vi "FA_ApplyINI.vi"(8 "Error In":errorcluster) -> (0 "Error Out":errorcluster)   [LabVIEW 2014, in "FA_INI.lvlib"]
doc: "Reads the XML file describing an INI configuration and applies the configuration to the target"
uses:
  FA_INI.lvlib
  FA_INIconfig.ctl
  FA_INI.ctl
  FA_LocalStore API/source/VI Source/FA_LSSpecialTypes.ctl
  FA_LocalStore API/source/VI Source/FA_LocalStore.lvlib
panel:
  out "Config":T1
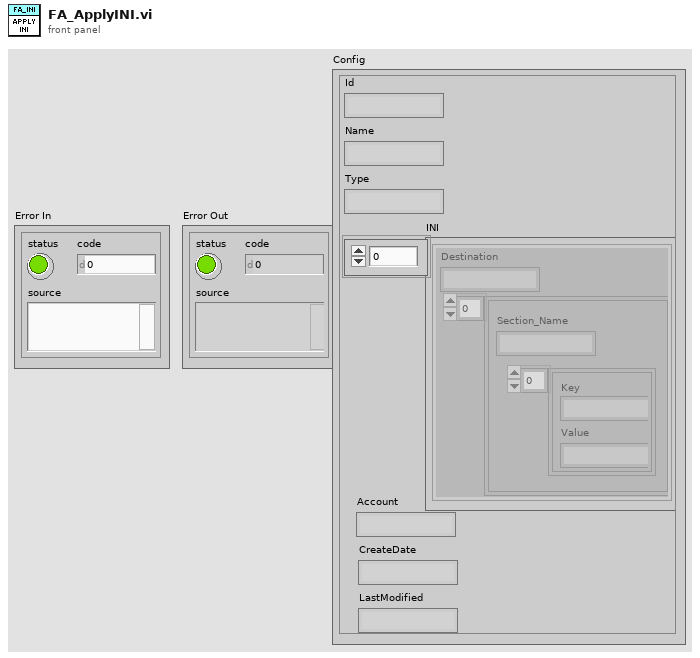
[diagram p1: front panel]
types:
  T1 = typedef "FA_INI.lvlib/FA_INIconfig.ctl" = cluster{"Id":string, "Name":string, "Type":string, "INI":T2, "Account":string, "CreateDate":string, "LastModified":string}
  T2 = typedef "FA_INI.ctl" = cluster{"Destination":string, "Section":cluster{"Section_Name":string, "Token":cluster{"Key":string, "Value":string}[]}[]}[]
  T3 = typedef "FA_LocalStore.lvlib/FA_LSSpecialTypes.ctl" = string
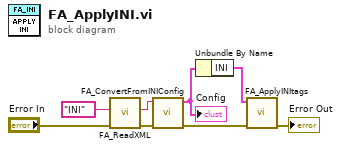
[diagram p0: block diagram]
diagram:
  n1 = call "FA_ReadXML.vi"("Error In"="Error In", "Special Type"=T3 "INI") -> ("Error Out"=w4:errorcluster, "XML String"=w2:string)  [unwired: 6 in]
  n2 = call "FA_ConvertFromINIConfig.vi"("Error In"=w4, "XML String"=w2) -> ("Error Out"=w6:errorcluster, "Config"=w8:T1)  [unwired: 8 in]
  "Config" <- w8
  n3 = Unbundle By Name(w8) -> ("INI"=w7:T2)
  n4 = call "FA_ApplyINItags.vi"("error in (no error)"=w6, "INI"=w7) -> ("error out"=→"Error Out":errorcluster)  [unwired: 9 in]
